vi "fisiere_v2.vi"() -> ()   [LabVIEW 2009]
panel:
  out "Citire din fisier terminata":bool
  out "Tari si capitale":string[][](array[string])
  in  "Selectati calea si fisierul":path=path "E:/Projects/Lab_view/Vi/fisiere/country-capital.txt"
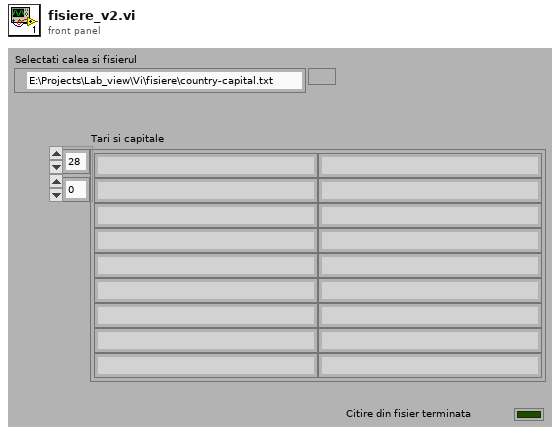
[diagram p1: front panel]
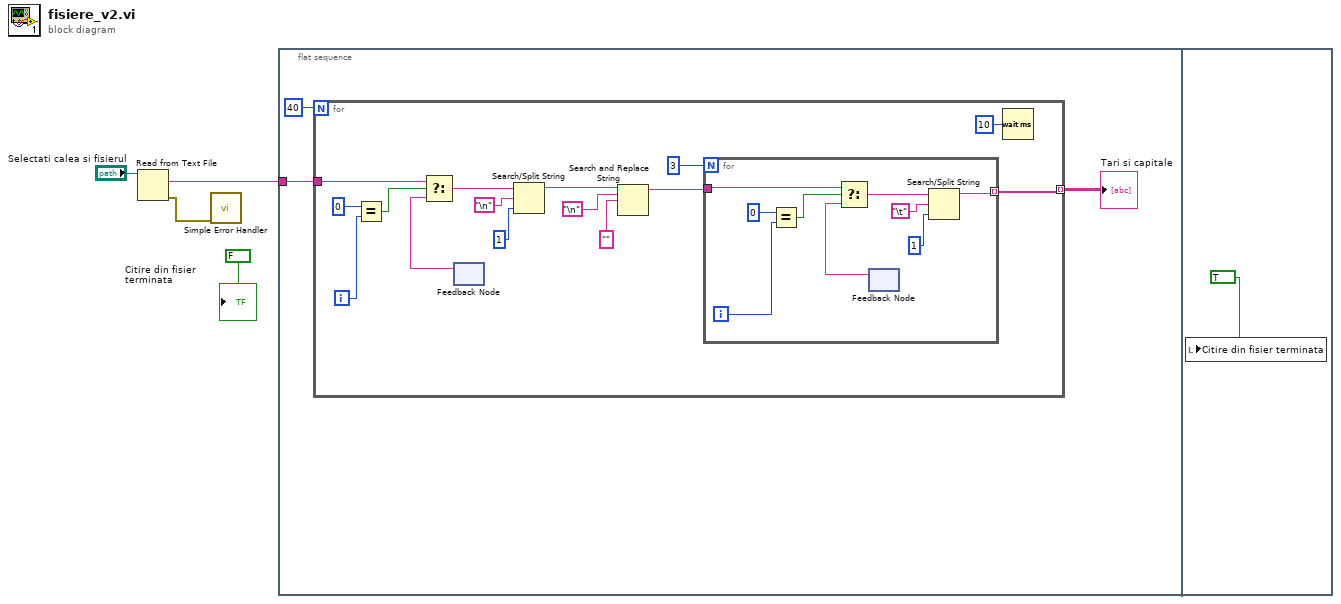
[diagram p0: block diagram]
diagram:
  n1 = Read from Text File(file (use dialog)="Selectati calea si fisierul") -> (text=w3:string, error out=w2:errorcluster)  [unwired: 3 in, 2 out]
  n2 = call <vilib>:"Simple Error Handler.vi"("error in (no error)"=w2) -> ()  [unwired: 4 in, 5 out]
  n3 = flat-sequence {
    tunnel: w3 -> [w7]
    frame #0 {
      n4 = for {
        N: 40 -> [_]
        tunnel: w7 -> [w20]
        tunnel: [w9] -> w5 mode=indexing
        i -> [w19]
        n5 = Equal?(x=0, y=w19) -> (x = y?=w17:bool)
        n6 = feedback #1() -> (w21:string)  [unwired: 1 in]
        n7 = Select(t=w20, s=w17, f=w21) -> (s? t:f=w16:string)
        n8 = Search/Split String(string=w16, search string/char (-)="\n", offset (0)=1) -> (substring before match=w14:string, match + rest of string=w15:string)  [unwired: 1 out]
        n9 = Search and Replace String(input string=w14, search string="\n", replace string="") -> (result string=w10:string)  [unwired: 5 in, 3 out]
        n10 = for {
          N: 3 -> [_]
          tunnel: w10 -> [w25]
          tunnel: [w24] -> w9 mode=indexing
          i -> [w26]
          n11 = Equal?(x=0, y=w26) -> (x = y?=w29:bool)
          n12 = feedback #2() -> (w31:string)  [unwired: 1 in]
          n13 = Select(t=w25, s=w29, f=w31) -> (s? t:f=w28:string)
          n14 = Search/Split String(string=w28, search string/char (-)="\t", offset (0)=1) -> (substring before match=w24:string, match + rest of string=w27:string)  [unwired: 1 out]
        }
        n15 = Wait (ms)(milliseconds to wait=u32 10) -> ()  [unwired: 1 out]
      }
      "Tari si capitale" <- w5
    }
    frame #1 {
      n16 = local write "Citire din fisier terminata"(TRUE ("Ready")) -> ()
    }
  }
  "Citire din fisier terminata" <- FALSE ("Af_start")
